vi "Create Scan.vi"(6 "Post action (indexing priority)":T1=[enum."Do Nothing", enum."Wait (Temperature)", enum."Do Nothing", enum."Do Nothing"], 9 "Scan parameters":T3=[{"Start"=0.14, "End"=-0.060000000000000005, "Step"=-0.060000000000000005, "Rate"=0.0, "Waveform type"=enum."linear", "wait (ms or K)"=10000.0, "Address"="Dev2/ao0", "channel"=1}, {"Start"=0.14, "End"=-0.060000000000000005, "Step"=-0.060000000000000005, "Rate"=0.0, "Waveform type"=enum."linear", "wait (ms or K)"=10000.0, "Address"="Dev2/ao0", "channel"=1}, {"Start"=0.14, "End"=-0.060000000000000005, "Step"=-0.060000000000000005, "Rate"=0.0, "Waveform type"=enum."linear", "wait (ms or K)"=10000.0, "Address"="Dev2/ao0", "channel"=1}, {"Start"=0.14, "End"=-0.060000000000000005, "Step"=-0.060000000000000005, "Rate"=0.0, "Waveform type"=enum."linear", "wait (ms or K)"=10000.0, "Address"="Dev2/ao0", "channel"=1}] {"Rate" format="%.2f"; "Step" format="%#_6p"; "End" format="%#_6p"; "Start" format="%#_6p"}, 10 "Scan control":T5=[{"Priority"=enum."Priority 1", "Scan name"=enum."Lockin Amplitude"}, {"Priority"=enum."Priority 2", "Scan name"=enum."Lockin Bias"}, {"Priority"=enum."Priority 0", "Scan name"=enum."Delay"}, {"Priority"=enum."Priority 2", "Scan name"=enum."Magnet Field"}], 11 "SweepControl":refnum<class "SweepControl.lvclass">) -> (3 "SweepControl":refnum<class "SweepControl.lvclass">)   [LabVIEW 2016, in "SweepControl.lvclass"]
uses:
  SweepControl.lvclass
  Typedefs/Cluster - ScanControl.ctl
  Typedefs/ScanControl.ctl
  Typedefs/Cluster - ScanParamters.ctl
  Typedefs/ScanParamters.ctl
  Typedefs/Enum - Priority.ctl
  Typedefs/Enum - Action.ctl
  Typedefs/Enum - PostAction.ctl
  Typedefs/PostAction.ctl
panel:
  out "error out":errorcluster
  in  "error in (no error)":errorcluster
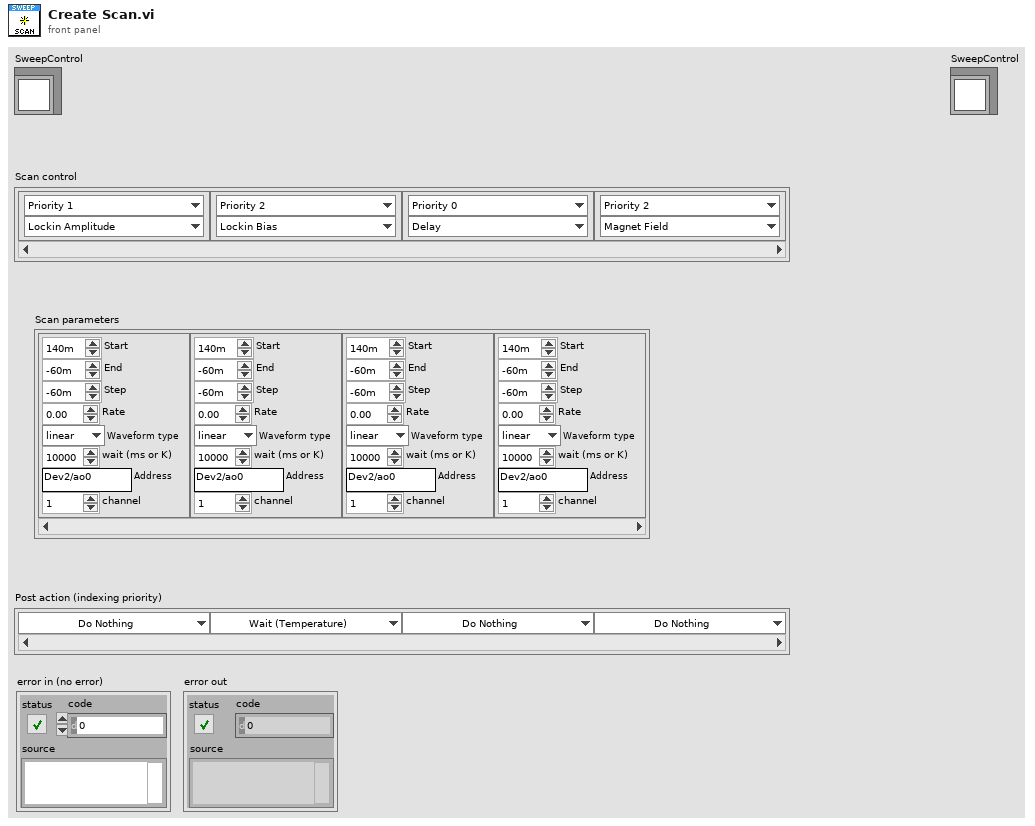
[diagram p1: front panel]
types:
  T1 = typedef "SweepControl.lvclass/PostAction.ctl" = T2[]
  T2 = typedef "SweepControl.lvclass/Enum - PostAction.ctl" = enum16{"Do Nothing", "Wait (time)", "Wait (Temperature)", "Wait (<T ; B sweep)", "Wait (Magnet)"}
  T3 = typedef "SweepControl.lvclass/ScanParamters.ctl" = T4[]
  T4 = typedef "SweepControl.lvclass/Cluster - ScanParamters.ctl" = cluster{"Start":dbl, "End":dbl, "Step":dbl, "Rate":dbl, "Waveform type":enum16{"linear", "triangle", "power"}, "wait (ms or K)":dbl, "Address":string, "channel":i32}
  T5 = typedef "SweepControl.lvclass/ScanControl.ctl" = T6[]
  T6 = typedef "SweepControl.lvclass/Cluster - ScanControl.ctl" = cluster{"Priority":T7, "Scan name":T8}
  T7 = typedef "SweepControl.lvclass/Enum - Priority.ctl" = enum16{"Priority 0", "Priority 1", "Priority 2", "Priority 3", "Priority 4", "Priority 5"}
  T8 = typedef "SweepControl.lvclass/Enum - Action.ctl" = enum16{"OFF", "time", "Lockin Amplitude", "Lockin Frequency", "Lockin Bias", "Delay", "Strain", "DAQ Bias", "Magnet Field", "Temperature", "MW f1", "MW f2", "MW Amplitude1", "MW Amplitude2"}
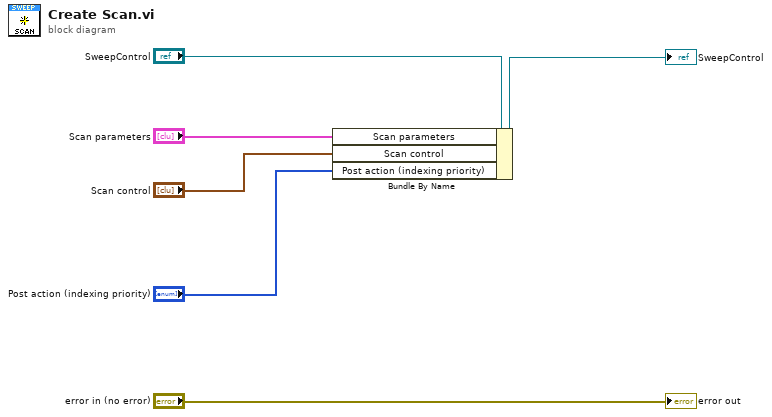
[diagram p0: block diagram]
diagram:
  n1 = Bundle By Name(cluster="SweepControl", "Scan parameters"="Scan parameters", "Scan control"="Scan control", "Post action (indexing priority)"="Post action (indexing priority)") -> (→"SweepControl":refnum<class "SweepControl.lvclass">)
  "error out" <- "error in (no error)"
